vi "Default Surface Property.vi"(11 "Plot ID":i32) -> (3 "Default Property":T1={"General Property"={"Plot Name"="", "Coordinate System"=enum."Cartesian", "Opacity"=0.0}, "Projection Property"={"Draw XY"=FALSE, "Draw YZ"=FALSE, "Draw XZ"=FALSE}, "Plot Property"={"Draw Surface"=FALSE, "Draw Mesh"=FALSE, "Draw Normal"=FALSE, "Color Ramp Cluster"={"Color Ramp Style"=enum."None", "Color Ramp Array"=[16711934, 393471, 57855, 4390754, 16449346, 16744722, 16711680], "Color Ramp Index"=[45, 91, 133, 175, 219, 255], "Interpolate?"=FALSE, "Logarithm?"=FALSE}, "Line Style"=enum."None", "Line Width"=0.0, "Line Color"=0, "Antialiasing"=FALSE}, "Surface Property"={"Color Mode"=enum."Flat Shading"}})   [LabVIEW 2020, in "3D Surface.lvclass"]
uses:
  3D Surface.lvclass
  3D Surface Property.ctl
  Color Ramp Cluster.ctl
  Line Type.ctl
  3D Plot.lvclass
panel:
  in  "Name Prefix":string="Plot "
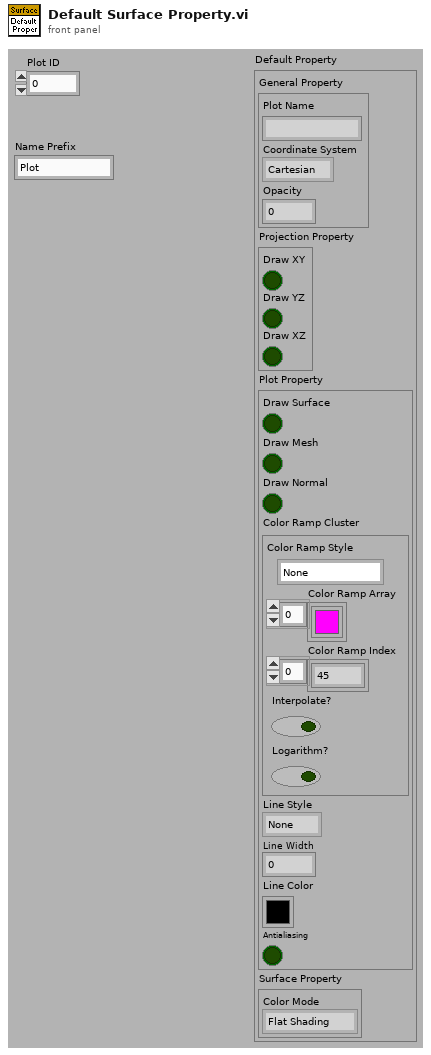
[diagram p1: front panel]
types:
  T1 = typedef "3D Surface.lvclass/3D Surface Property.ctl" = cluster{"General Property":cluster{"Plot Name":string, "Coordinate System":enum16{"Cartesian", "Cylindrical", "Spherical"}, "Opacity":sgl}, "Projection Property":cluster{"Draw XY":bool, "Draw YZ":bool, "Draw XZ":bool}, "Plot Property":cluster{"Draw Surface":bool, "Draw Mesh":bool, "Draw Normal":bool, "Color Ramp Cluster":T2, "Line Style":T3, "Line Width":sgl, "Line Color":u32, "Antialiasing":bool}, "Surface Property":cluster{"Color Mode":enum16{"Flat Shading", "Interpolated Shading"}}}
  T2 = typedef "3D Plot.lvclass/Color Ramp Cluster.ctl" = cluster{"Color Ramp Style":enum16{"None", "Shaded", "Color spectrum", "Grey scale", "Custom"}, "Color Ramp Array":u32[], "Color Ramp Index":i32[], "Interpolate?":bool, "Logarithm?":bool}
  T3 = typedef "3D Plot.lvclass/Line Type.ctl" = enum16{"None", "Solid", "Dash", "Dot", "Dash Dot"}
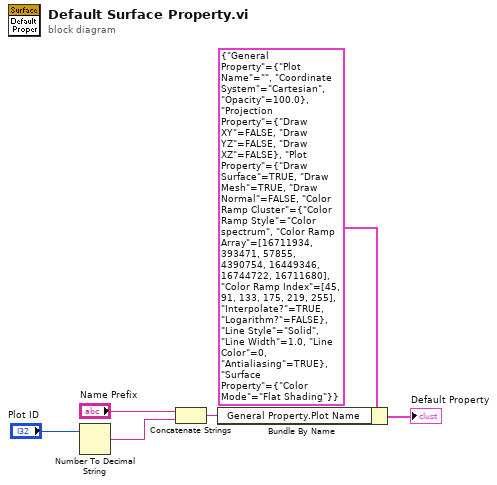
[diagram p0: block diagram]
diagram:
  n1 = Number To Decimal String(number="Plot ID") -> (decimal integer string=w3:string)  [unwired: 1 out]
  n2 = Concatenate Strings("Name Prefix", w3) -> (w6:string)
  n3 = Bundle By Name(cluster=T1 {"General Property"={"Plot Name"="", "Coordinate System"=enum."Cartesian", "Opacity"=100.0}, "Projection Property"={"Draw XY"=FALSE, "Draw YZ"=FALSE, "Draw XZ"=FALSE}, "Plot Property"={"Draw Surface"=TRUE, "Draw Mesh"=TRUE, "Draw Normal"=FALSE, "Color Ramp Cluster"={"Color Ramp Style"=enum."Color spectrum", "Color Ramp Array"=[16711934, 393471, 57855, 4390754, 16449346, 16744722, 16711680], "Color Ramp Index"=[45, 91, 133, 175, 219, 255], "Interpolate?"=TRUE, "Logarithm?"=FALSE}, "Line Style"=enum."Solid", "Line Width"=1.0, "Line Color"=0, "Antialiasing"=TRUE}, "Surface Property"={"Color Mode"=enum."Flat Shading"}} ("new element/subarray"), "General Property.Plot Name"=w6) -> (→"Default Property":T1)
